vi "XY_sequence_generator.vi"(10 "Acquisition time (ms)":dbl, 11 "XY acquisition":T1={"Number of tiles in X"=3.0, "Number of tiles in Y"=3.0, "Step size XY (µm)"=500.0, "Acquire XY-tiling"=FALSE, "Moving time (ms)"=1000.0}) -> (3 "string array":string[](array[string]))   [LabVIEW 2020]
uses:
  typedefs/typedef_XY_tiling.ctl
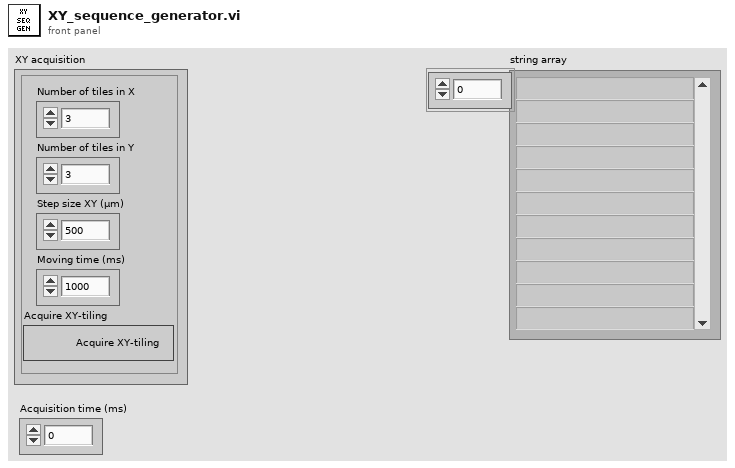
[diagram p1: front panel]
types:
  T1 = typedef "typedef_XY_tiling.ctl" = cluster{"Number of tiles in X":dbl, "Number of tiles in Y":dbl, "Step size XY (µm)":dbl, "Acquire XY-tiling":bool, "Moving time (ms)":dbl}
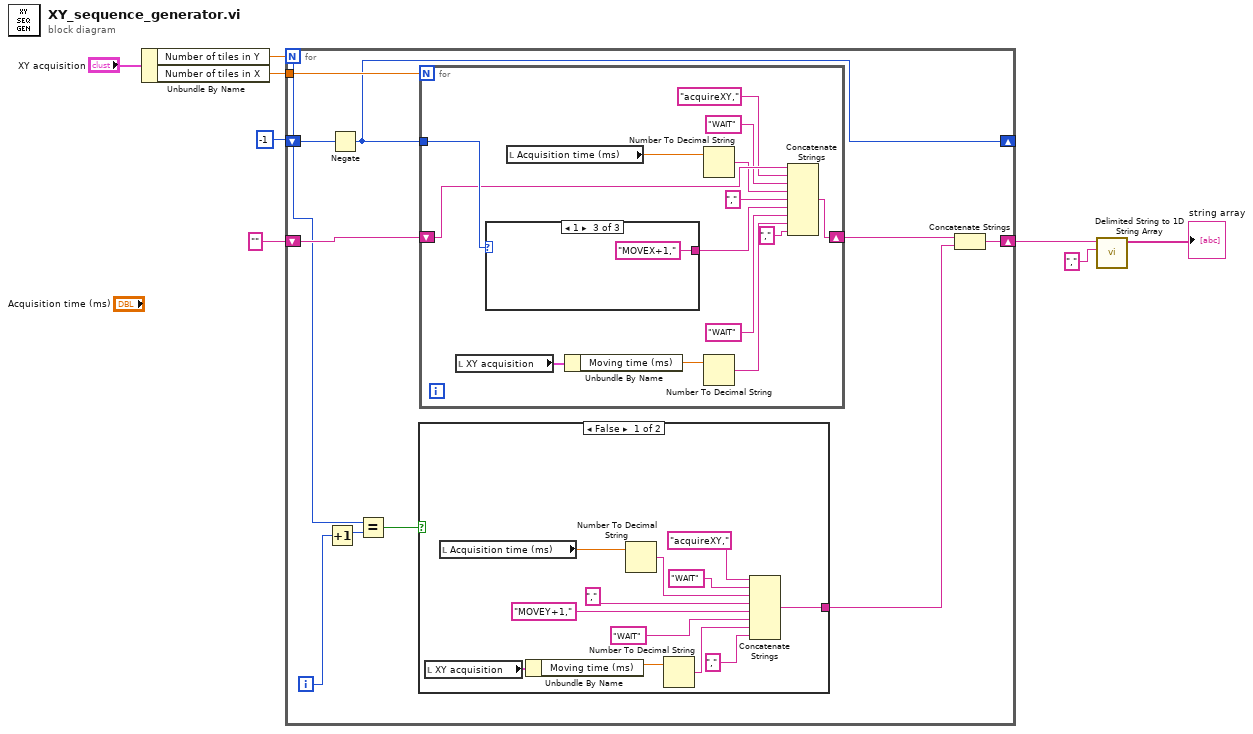
[diagram p0: block diagram]
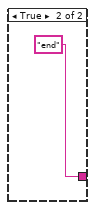
[diagram p2: hidden frame]
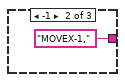
[diagram p4: hidden frame]
diagram:
  n1 = Unbundle By Name("XY acquisition") -> ("Number of tiles in Y"=w1:dbl, "Number of tiles in X"=w2:dbl)
  n2 = for {
    N: w1 -> [w12]
    tunnel: w2 -> [w19]
    shift-right: [w14] -> _
    shift-left: -1 -> [w15]
    shift-right: [w16] -> w5
    shift-left: "" -> [w18]
    i -> [w9]
    n3 = Increment(x=w9) -> (x+1=w10:i32)
    n4 = Negate(x=w15) -> (-x=w14:i32)
    n5 = Equal?(x=w12, y=w10) -> (x = y?=w13:bool)
    n6 = case shown="False" w13 {
      tunnel: [w27 "end" ("string")] -> w11
      frame False {
        n7 = local read "XY acquisition"() -> (w28:T1)
        n8 = local read "Acquisition time (ms)"() -> (w20:dbl)
        n9 = Unbundle By Name(w28) -> ("Moving time (ms)"=w30:dbl)
        n10 = Number To Decimal String(number=w20) -> (decimal integer string=w23:string)  [unwired: 1 in]
        n11 = Number To Decimal String(number=w30) -> (decimal integer string=w29:string)  [unwired: 1 in]
        n12 = Concatenate Strings("acquireXY," ("string"), "WAIT" ("string"), w23, "," ("string"), "MOVEY+1," ("string"), "WAIT" ("string"), w29, "," ("string")) -> (w27:string)
      }
      frame True {
      }
    }
    n13 = for {
      N: w19 -> [_]
      tunnel: w14 -> [w44]
      shift-right: [w45] -> w17
      shift-left: w18 -> [w38]
      n14 = local read "XY acquisition"() -> (w42:T1)
      n15 = case shown="1" w44 {
        tunnel: [_ "MOVEX-1," "MOVEX+1,"] -> w46
        frame 0, Default {
        }
        frame -1 {
        }
        frame 1 {
        }
      }
      n16 = local read "Acquisition time (ms)"() -> (w33:dbl)
      n17 = Unbundle By Name(w42) -> ("Moving time (ms)"=w40:dbl)
      n18 = Number To Decimal String(number=w33) -> (decimal integer string=w35:string)  [unwired: 1 in]
      n19 = Number To Decimal String(number=w40) -> (decimal integer string=w41:string)  [unwired: 1 in]
      n20 = Concatenate Strings(w38, "acquireXY," ("string"), "WAIT" ("string"), w35, "," ("string"), w46, "WAIT" ("string"), w41, "," ("string")) -> (w45:string)
    }
    n21 = Concatenate Strings(w17, w11) -> (w16:string)
  }
  n22 = call <vilib>:"Delimited String to 1D String Array.vi"("delimiter"=",", "delimited string"=w5) -> ("string array"=→"string array":string[])  [unwired: 9 in]
